vi "Select Self Test Bus Channels.vi"(7 "Channels":i32[](array[numeric])) -> (8 "Selected Channels":i32[](array[numeric]))   [LabVIEW 2020]
panel:
  in  "Rx":cluster{"Boolean":string, "Enable":bool}[](array[cluster])
  in  "Continue Button":bool
  in  "Tx":cluster{"Boolean":string, "Enable":bool}[](array[cluster])
  # "Select the channels you would like to connect to the internal self test bus."
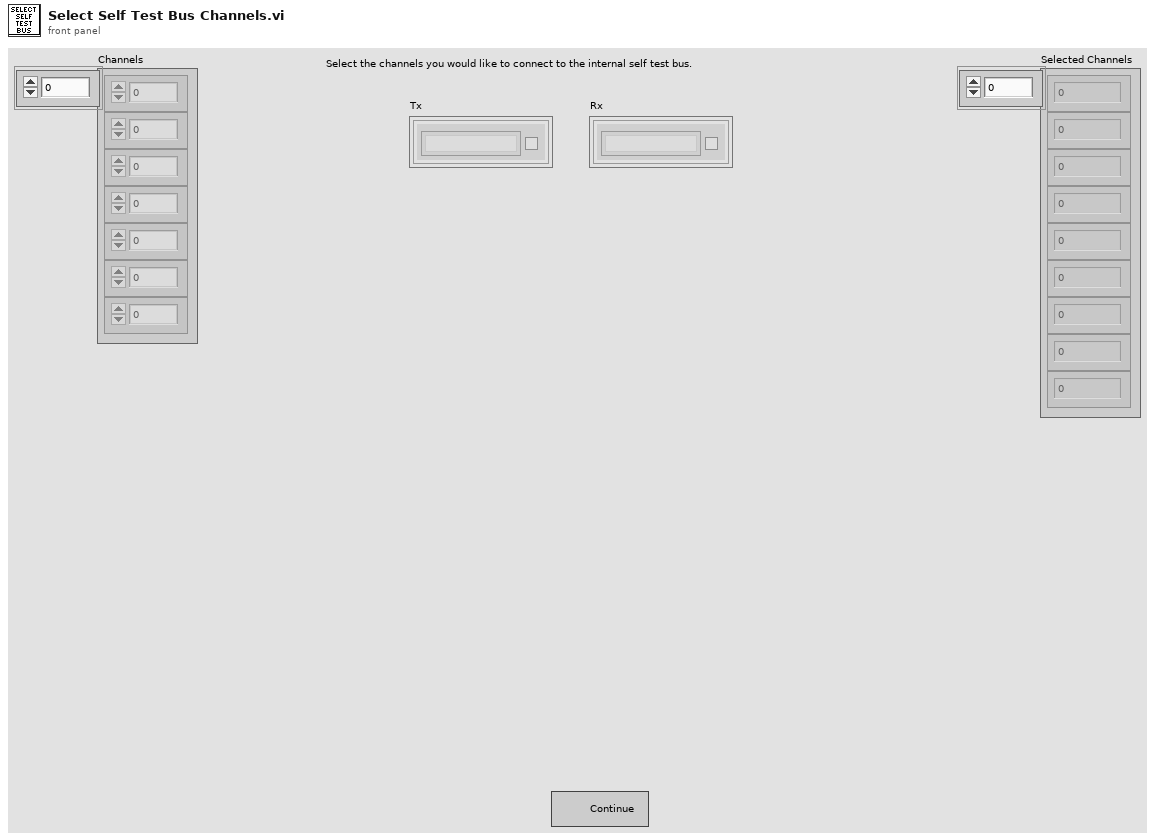
[diagram p1: front panel]
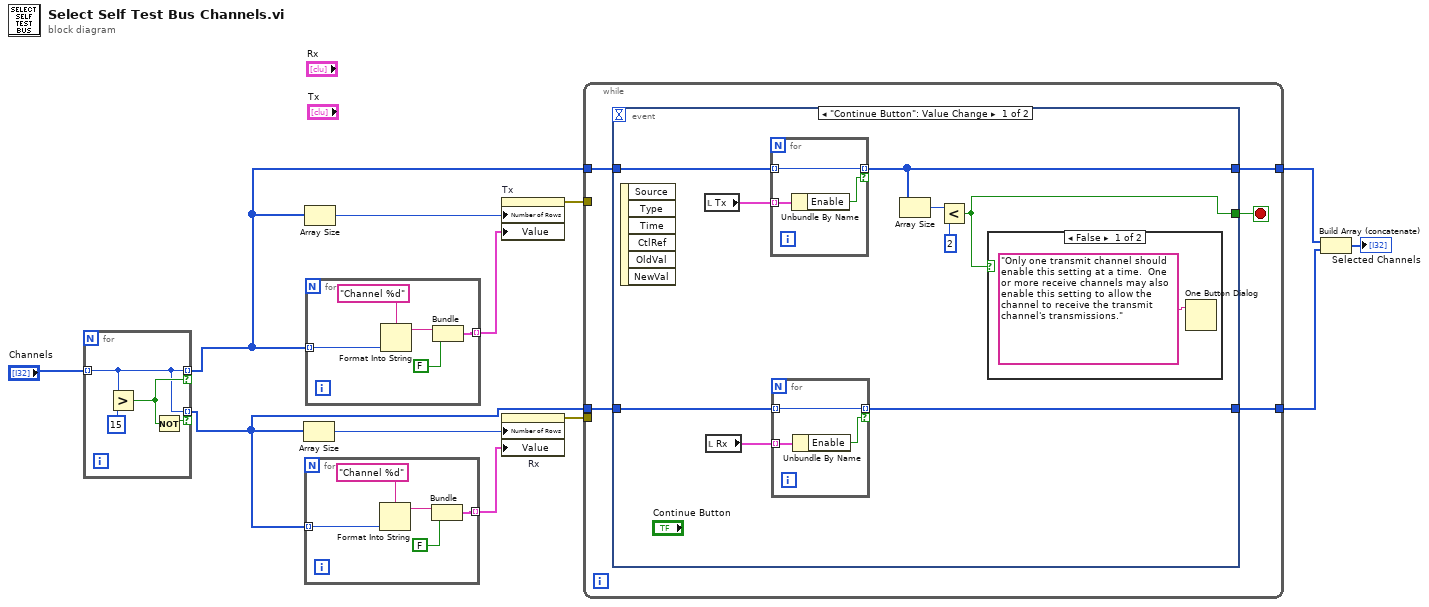
[diagram p0: block diagram]
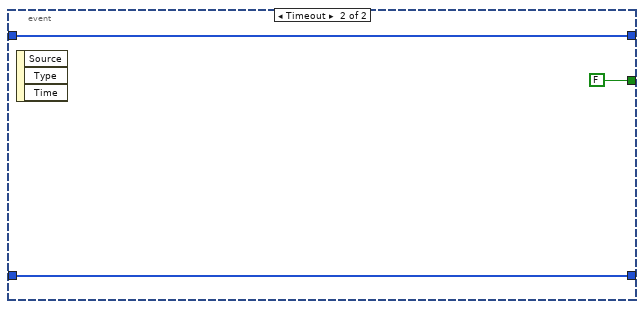
[diagram p3: hidden frame]
diagram:
  n1 = for {
    tunnel: "Channels" -> [w14] mode=indexing
    tunnel: [w14] -> w5 mode=indexing if=w15
    tunnel: [w14] -> w4 mode=indexing if=w13
    n2 = Greater?(x=w14, y=15) -> (0:w15:bool)
    n3 = Not(x=w15) -> (.not. x?=w13:bool)
  }
  n4 = Array Size(array=w4) -> (size(s)=w8:i32)
  n5 = Array Size(array=w5) -> (size(s)=w9:i32)
  n6 = for {
    tunnel: w4 -> [w21] mode=indexing
    tunnel: [w17] -> w7 mode=indexing
    n7 = Format Into String(format string="Channel %d", w21) -> (resulting string=w19:string)  [unwired: 2 in, 1 out]
    n8 = Bundle(w19, FALSE) -> (w17:cluster{string, bool})  [unwired: 1 in]
  }
  n9 = for {
    tunnel: w5 -> [w26] mode=indexing
    tunnel: [w22] -> w11 mode=indexing
    n10 = Format Into String(format string="Channel %d", w26) -> (resulting string=w24:string)  [unwired: 2 in, 1 out]
    n11 = Bundle(w24, FALSE) -> (w22:cluster{string, bool})  [unwired: 1 in]
  }
  n12 = property on="Tx" class="Arr (strict)"("Number of Rows"=w9, "Value"=w11) -> (error out=w10:errorcluster)  [unwired: 2 in, 1 out]
  n13 = property on="Rx" class="Arr (strict)"("Number of Rows"=w8, "Value"=w7) -> (error out=w6:errorcluster)  [unwired: 2 in, 1 out]
  n14 = while {
    tunnel: w10 -> [_]
    tunnel: w6 -> [_]
    tunnel: w5 -> [w31]
    tunnel: [w30] -> w3
    tunnel: w4 -> [w29]
    tunnel: [w28] -> w2
    stop <- w27 stop-if-true
    n15 = event shown="[0] \"Continue Button\": Value Change" {
      selector: _ -> [_ _]
      dyn-events: _ -> [_ _]
      timeout: _ -> [_ _]
      tunnel: w31 -> [w39 w49]
      tunnel: [w35 w49] -> w30
      tunnel: w29 -> [w37 w48]
      tunnel: [w36 w48] -> w28
      tunnel: [w32 FALSE] -> w27
      event "Continue Button": Value Change {
        n16 = event-data() -> ()  [unwired: 1 in, 6 out]
        n17 = local read "Tx"() -> (w40:cluster{"Boolean":string, "Enable":bool}[])
        n18 = local read "Rx"() -> (w38:cluster{"Boolean":string, "Enable":bool}[])
        n19 = for {
          tunnel: w40 -> [w46] mode=indexing
          tunnel: w39 -> [w47] mode=indexing
          tunnel: [w47] -> w35 mode=indexing if=w45
          n20 = Unbundle By Name(w46) -> ("Enable"=w45:bool)
        }
        n21 = for {
          tunnel: w38 -> [w43] mode=indexing
          tunnel: w37 -> [w44] mode=indexing
          tunnel: [w44] -> w36 mode=indexing if=w42
          n22 = Unbundle By Name(w43) -> ("Enable"=w42:bool)
        }
        n23 = Array Size(array=w35) -> (size(s)=w34:i32)
        n24 = Less?(x=w34, y=2) -> (x < y?=w32:bool)
        n25 = case shown="False" w32 {
          frame False {
            n26 = One Button Dialog(message="Only one transmit channel should enable this setting at a time.  One or more receive channels may also enable this setting to allow the channel to receive the transmit channel's transmissions.") -> ()  [unwired: 1 in, 1 out]
          }
          frame True {
          }
        }
      }
      event Timeout {
        n27 = event-data() -> ()  [unwired: 1 in, 3 out]
      }
    }
  }
  n28 = Build Array (concatenate)(w3, w2) -> (→"Selected Channels":i32[])
